vi "Periodic Tasks.vi"(8 "error in":errorcluster) -> ()   [LabVIEW 2012]
doc: "This VI runs in parallel to other tasks. It can contain as many user-defined periodic loops as you need. These can carry out PID or other sorts of timed response."
uses:
  <vilib>/Rock Robotics/SystemInterfaces/Utilities/FPGA_UtilitiesLED Source.ctl
  <vilib>/Rock Robotics/SystemInterfaces/Utilities/FPGA_UtilitiesLED State.ctl
  <vilib>/Rock Robotics/WPI/Compressor/WPI_CompressorGetSetRefNum.vi
  Robot Global Data.vi
  <vilib>/Rock Robotics/WPI/Joystick/WPI_JoystickGetSetRefNum.vi
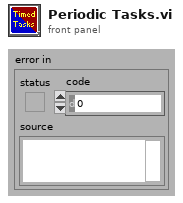
[diagram p1: front panel]
types:
  T1 = typedef "FPGA_UtilitiesLED State.ctl" = enum16{"Off", "On", "Toggle"}
  T2 = typedef "FPGA_UtilitiesLED Source.ctl" = enum16{"User LED", "FPGA LED"}
  T3 = typedef "WPI_CompressorDevRef.ctl" = cluster{"DevStatus":errorcluster, "DigitalInputDevRef":T4, "RelayDevRef":T7}
  T4 = typedef "WPI_DigitalInputDevRef.ctl" = cluster{"DevStatus":errorcluster, "DIO Channel":T5, "Digital Module":T6}
  T5 = typedef "FPGA_DIOChannel.ctl" = enum8{"DIO 1", "DIO 2", "DIO 3", "DIO 4", "DIO 5", "DIO 6", "DIO 7", "DIO 8", "DIO 9", "DIO 10", "DIO 11", "DIO 12", "DIO 13", "DIO 14", "Invalid"}
  T6 = typedef "FPGA_TypedefDigitalModule.ctl" = enum16{"Digital Module 1", "Digital Module 2"}
  T7 = typedef "WPI_RelayDevRef.ctl" = cluster{"DevStatus":errorcluster, "Relay Channel":T8, "Digital Module":T6, "Relay Direction":T9}
  T8 = typedef "FPGA_DIORelayChannel.ctl" = enum8{"Relay 1", "Relay 2", "Relay 3", "Relay 4", "Relay 5", "Relay 6", "Relay 7", "Relay 8", "Invalid"}
  T9 = typedef "WPI_RelayDirection.ctl" = enum16{"Both directions", "Forward only", "Reverse only"}
  T10 = typedef "WPI_JoystickDevRef.ctl" = cluster{"Device":T11}
  T11 = typedef "WPI_JoystickDeviceEnum.ctl" = enum16{"USB 1", "USB 2", "USB 3", "USB 4", "Kinect 1", "Kinect 2"}
  T12 = typedef "WPI_JoystickButtonState.ctl" = cluster{"Button 1":bool, "Button 2":bool, "Button 3":bool, "Button 4":bool, "Button 5":bool, "Button 6":bool, "Button 7":bool, "Button 8":bool, "Button 9":bool, "Button 10":bool, "Button 11":bool, "Button 12":bool}
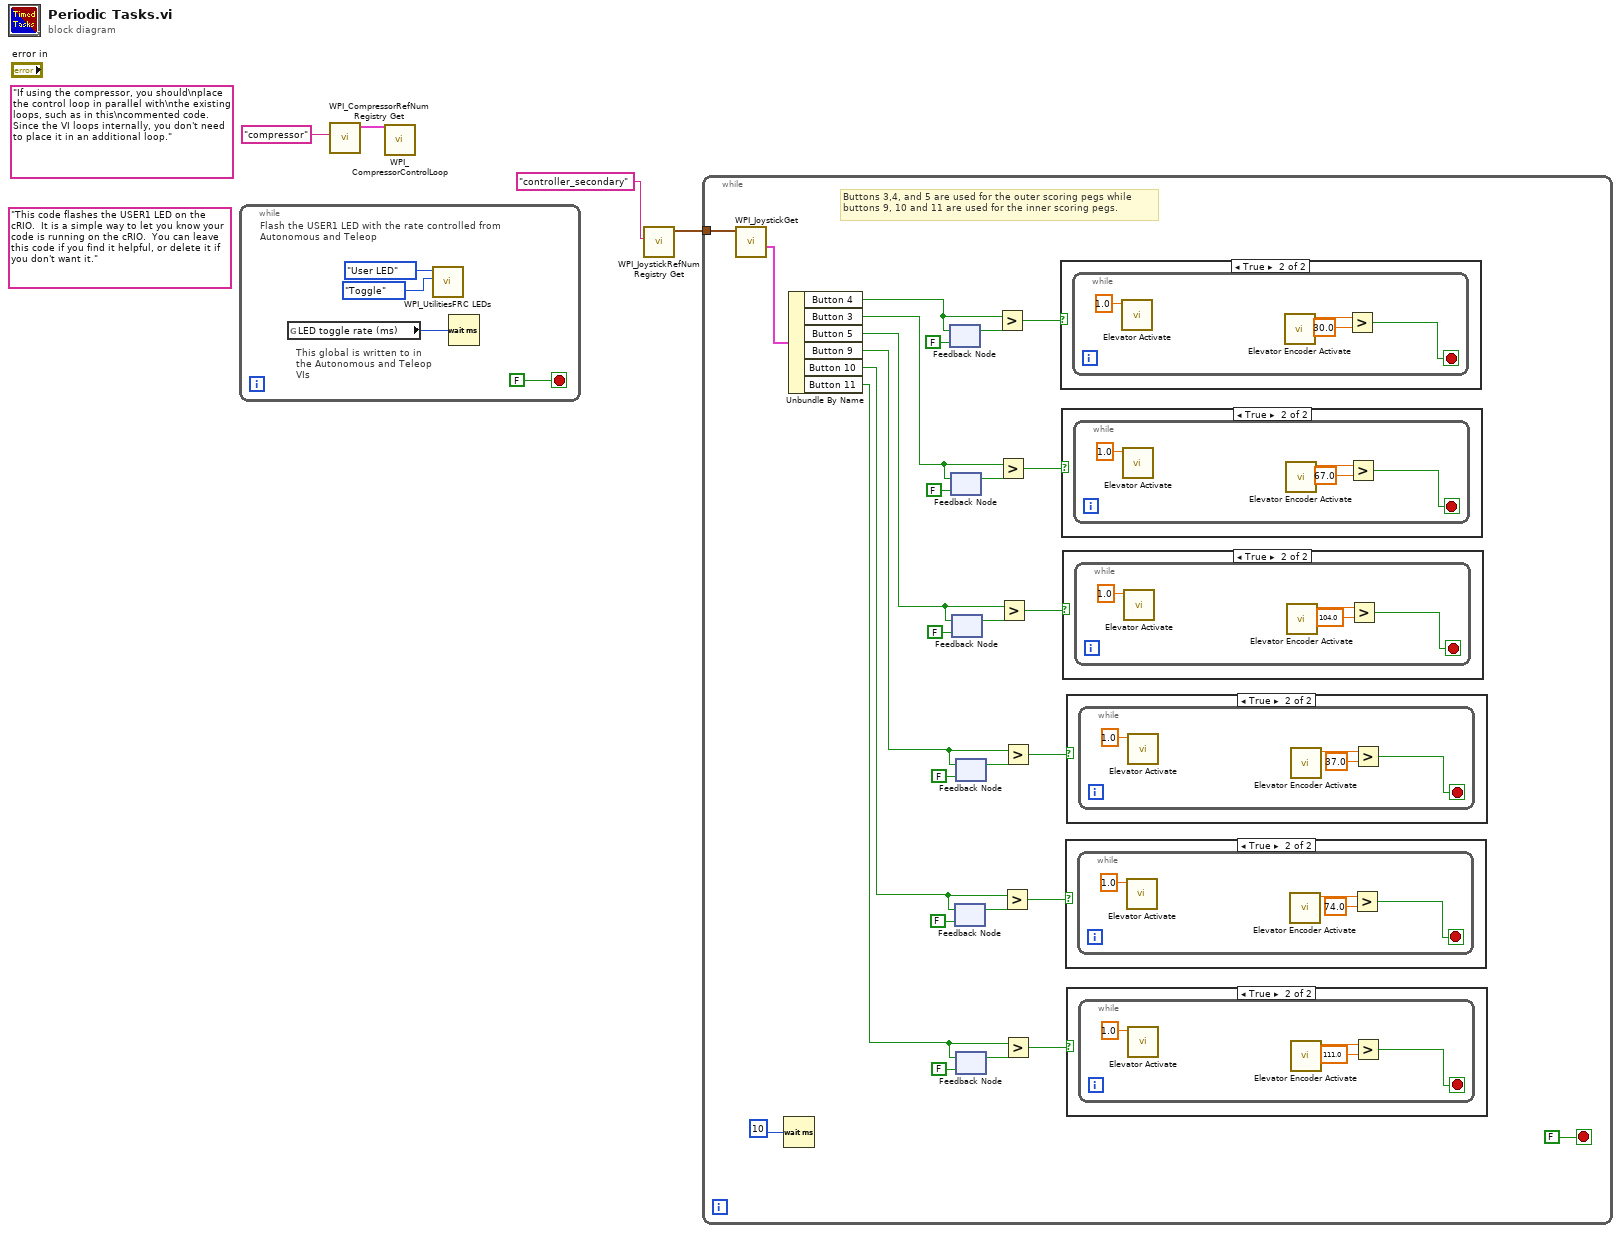
[diagram p0: block diagram]
diagram:
  (unwired) "If using the compressor, you should\nplace the control loop in parallel with\nthe existing loops, such as in this\ncommented code. Since the VI loops internally, you don't need to place it in an additional loop."
  (unwired) "This code flashes the USER1 LED on the cRIO.  It is a simple way to let you know your code is running on the cRIO.  You can leave this code if you find it helpful, or delete it if you don't want it."
  n1 = while {
    stop <- FALSE stop-if-true
    # "This global is written to in the Autonomous and Teleop VIs"
    # "Flash the USER1 LED with the rate controlled from Autonomous and Teleop"
    n2 = global read "Robot Global Data.vi" "LED toggle rate (ms)"() -> (w5:u32)
    n3 = call <vilib>:"WPI_UtilitiesFRC LEDs.vi"("State"=FPGA_UtilitiesLED_State."Toggle", "LED Type"=FPGA_UtilitiesLED_Source."User LED") -> ()  [unwired: 1 in, 9 out]
    n4 = Wait (ms)(milliseconds to wait=w5) -> ()  [unwired: 1 out]
  }
  n5 = call <vilib>:"WPI_CompressorRefNum Registry Get.vi"("refnum name"="compressor") -> ("CompressorDevRef"=w4:T3)  [unwired: 9 in, 1 out]
  n6 = call <vilib>:"WPI_CompressorControlLoop.vi"("CompressorDevRef"=w4) -> ()  [unwired: 11 in]
  n7 = call <vilib>:"WPI_JoystickRefNum Registry Get.vi"("refnum name"="controller_secondary") -> ("JoystickDevRef"=w1:T10)  [unwired: 9 in, 1 out]
  n8 = while {
    tunnel: w1 -> [w36]
    stop <- FALSE stop-if-true
    # "Buttons 3,4, and 5 are used for the outer scoring pegs while \nbuttons 9, 10 and 11 are used for the inner scoring pegs."
    n9 = call <vilib>:"WPI_JoystickGet.vi"("JoystickDevRef"=w36) -> ("Buttons"=w33:T12)  [unwired: 4 in, 2 out]
    n10 = Wait (ms)(milliseconds to wait=u32 10) -> ()  [unwired: 1 out]
    n11 = Unbundle By Name(w33) -> ("Button 4"=w26:bool, "Button 3"=w25:bool, "Button 5"=w21:bool, "Button 9"=w17:bool, "Button 10"=w13:bool, "Button 11"=w9:bool)
    n12 = feedback-in #1(w26) -> ()
    n13 = feedback #1(FALSE ("Button 2")) -> (w32:bool)
    n14 = feedback #2(FALSE ("Button 2")) -> (w27:bool)
    n15 = feedback-in #2(w25) -> ()
    n16 = feedback #3(FALSE ("Button 2")) -> (w22:bool)
    n17 = feedback-in #3(w21) -> ()
    n18 = feedback #4(FALSE ("Button 2")) -> (w14:bool)
    n19 = feedback-in #4(w13) -> ()
    n20 = feedback #5(FALSE ("Button 2")) -> (w20:bool)
    n21 = feedback-in #5(w17) -> ()
    n22 = feedback #6(FALSE ("Button 2")) -> (w12:bool)
    n23 = feedback-in #6(w9) -> ()
    n24 = Greater?(x=w26, y=w32) -> (0:w30:bool)
    n25 = Greater?(x=w25, y=w27) -> (0:w29:bool)
    n26 = Greater?(x=w21, y=w22) -> (0:w24:bool)
    n27 = Greater?(x=w13, y=w14) -> (0:w16:bool)
    n28 = Greater?(x=w17, y=w20) -> (0:w18:bool)
    n29 = Greater?(x=w9, y=w12) -> (0:w10:bool)
    n30 = case shown="True" w30 {
      frame False {
      }
      frame True {
        n31 = while {
          stop <- w58 stop-if-true
          n32 = call "Elevator Activate.vi"("Elevator Output"=1.0) -> ()  [unwired: 11 in]
          n33 = call "Elevator Encoder Activate.vi"() -> ("Distance"=w59:dbl)  [unwired: 11 in]
          n34 = Greater?(x=w59, y=30.0) -> (0:w58:bool)
        }
      }
    }
    n35 = case shown="True" w29 {
      frame False {
      }
      frame True {
        n36 = while {
          stop <- w54 stop-if-true
          n37 = call "Elevator Activate.vi"("Elevator Output"=1.0) -> ()  [unwired: 11 in]
          n38 = call "Elevator Encoder Activate.vi"() -> ("Distance"=w55:dbl)  [unwired: 11 in]
          n39 = Greater?(x=w55, y=67.0) -> (0:w54:bool)
        }
      }
    }
    n40 = case shown="True" w24 {
      frame False {
      }
      frame True {
        n41 = while {
          stop <- w50 stop-if-true
          n42 = call "Elevator Activate.vi"("Elevator Output"=1.0) -> ()  [unwired: 11 in]
          n43 = call "Elevator Encoder Activate.vi"() -> ("Distance"=w51:dbl)  [unwired: 11 in]
          n44 = Greater?(x=w51, y=104.0) -> (0:w50:bool)
        }
      }
    }
    n45 = case shown="True" w16 {
      frame False {
      }
      frame True {
        n46 = while {
          stop <- w42 stop-if-true
          n47 = call "Elevator Activate.vi"("Elevator Output"=1.0) -> ()  [unwired: 11 in]
          n48 = call "Elevator Encoder Activate.vi"() -> ("Distance"=w43:dbl)  [unwired: 11 in]
          n49 = Greater?(x=w43, y=74.0) -> (0:w42:bool)
        }
      }
    }
    n50 = case shown="True" w18 {
      frame False {
      }
      frame True {
        n51 = while {
          stop <- w46 stop-if-true
          n52 = call "Elevator Activate.vi"("Elevator Output"=1.0) -> ()  [unwired: 11 in]
          n53 = call "Elevator Encoder Activate.vi"() -> ("Distance"=w47:dbl)  [unwired: 11 in]
          n54 = Greater?(x=w47, y=37.0) -> (0:w46:bool)
        }
      }
    }
    n55 = case shown="True" w10 {
      frame False {
      }
      frame True {
        n56 = while {
          stop <- w38 stop-if-true
          n57 = call "Elevator Activate.vi"("Elevator Output"=1.0) -> ()  [unwired: 11 in]
          n58 = call "Elevator Encoder Activate.vi"() -> ("Distance"=w39:dbl)  [unwired: 11 in]
          n59 = Greater?(x=w39, y=111.0) -> (0:w38:bool)
        }
      }
    }
  }
